vi "Finalize Logger.vi"(8 "error in":errorcluster, 11 "Log Producer in":T1) -> (0 "error out":errorcluster, 3 "Log Producer out":T1)   [LabVIEW 2020, in "Frame Logging.lvlib"]
uses:
  Frame Logging.lvlib
  Message_Request_Action.ctl
  Message_Request.ctl
  Log_Producer.ctl
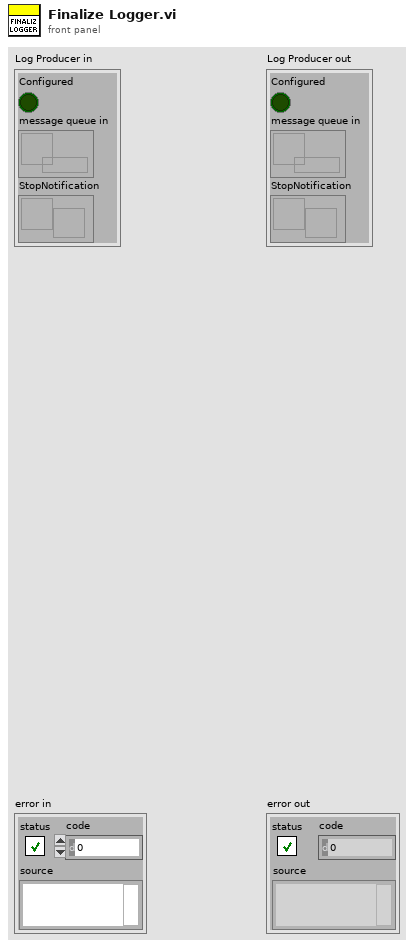
[diagram p1: front panel]
types:
  T1 = typedef "Frame Logging.lvlib/Log_Producer.ctl" = cluster{"Configured":bool, "message queue in":refnum<queue>, "StopNotification":refnum<notifier>}
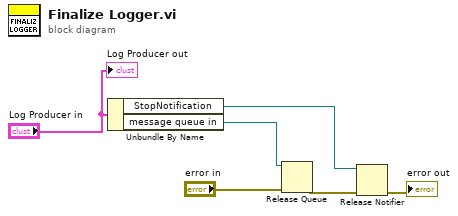
[diagram p0: block diagram]
diagram:
  n1 = Unbundle By Name("Log Producer in") -> ("StopNotification"=w1:refnum<notifier>, "message queue in"=w4:refnum<queue>)
  n2 = Release Queue(queue=w4, error in (no error)="error in") -> (error out=w3:errorcluster)  [unwired: 1 in, 2 out]
  n3 = Release Notifier(notifier=w1, error in (no error)=w3) -> (error out=→"error out":errorcluster)  [unwired: 1 in, 2 out]
  "Log Producer out" <- "Log Producer in"
